vi "EEG_FFT_Analyzer.vi"() -> ()   [LabVIEW 2014]
uses:
  <vilib>/DAQmx/create/channels.llb/DAQmx Create Channel (AI-Voltage-Basic).vi
  <vilib>/DAQmx/configure/timing.llb/DAQmx Timing (Sample Clock).vi
  <vilib>/DAQmx/read.llb/DAQmx Read (Analog 1D Wfm NChan NSamp).vi
panel:
  out "Beta_Power vs. Time":dbl[](graph)
  out "Alpha_Power vs. Time":dbl[](graph)
  out "Waveform of Selected EEG":dbl[](graph)
  in  "P4":bool
  in  "P3":bool
  in  "Pz":bool
  in  "O2":bool
  in  "O1":bool
  in  "C4":bool
  in  "C3":bool
  in  "Cz":bool
  in  "F4":bool
  in  "Fz":bool
  in  "F3":bool
  in  "stop":bool
  # "NASION"
  # "INION"
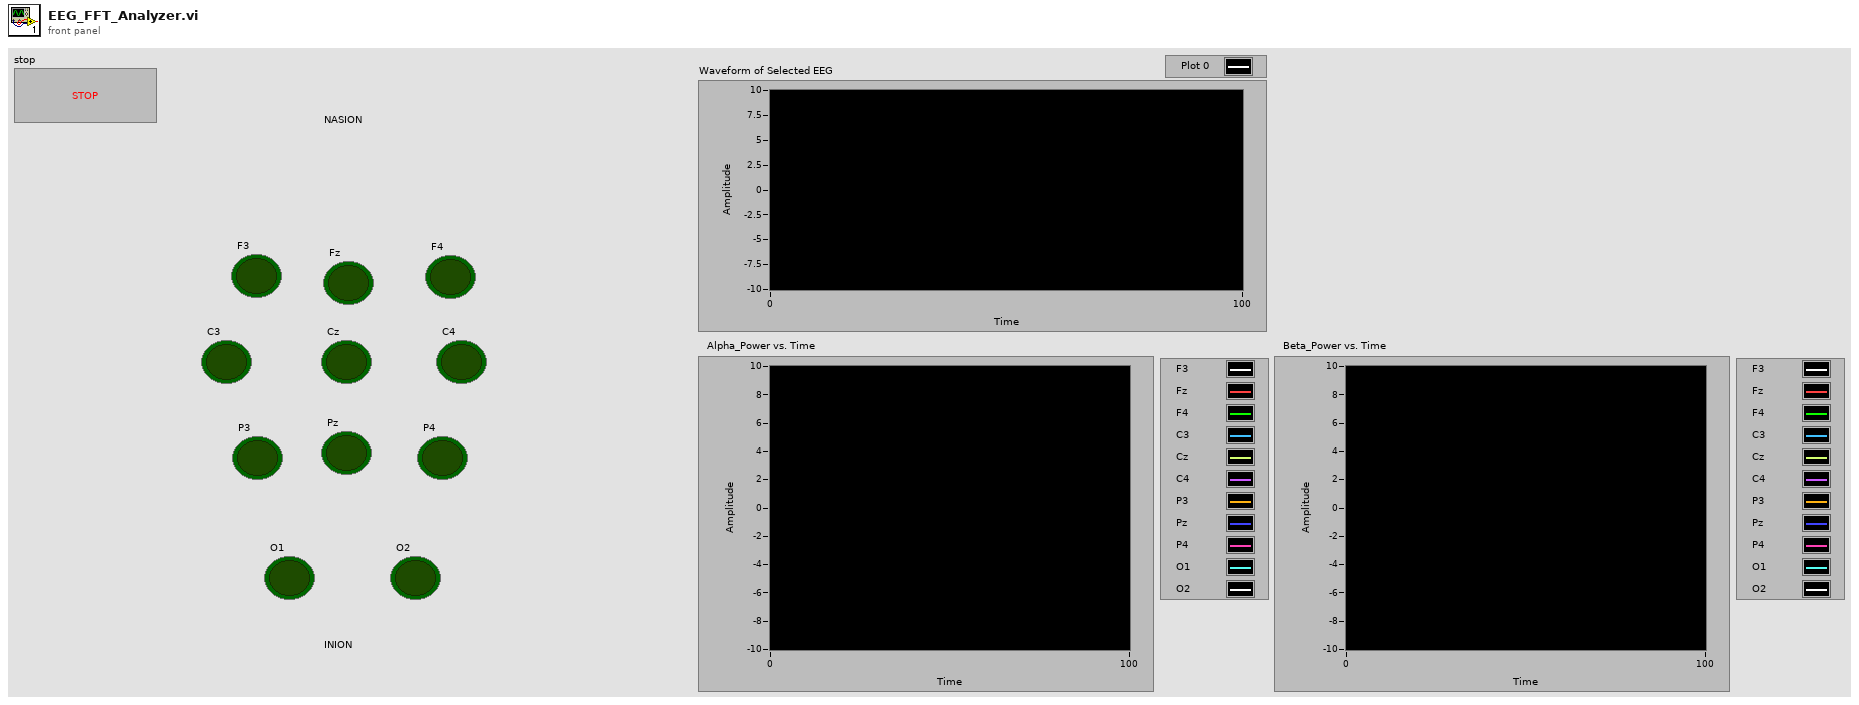
[diagram p1: front panel]
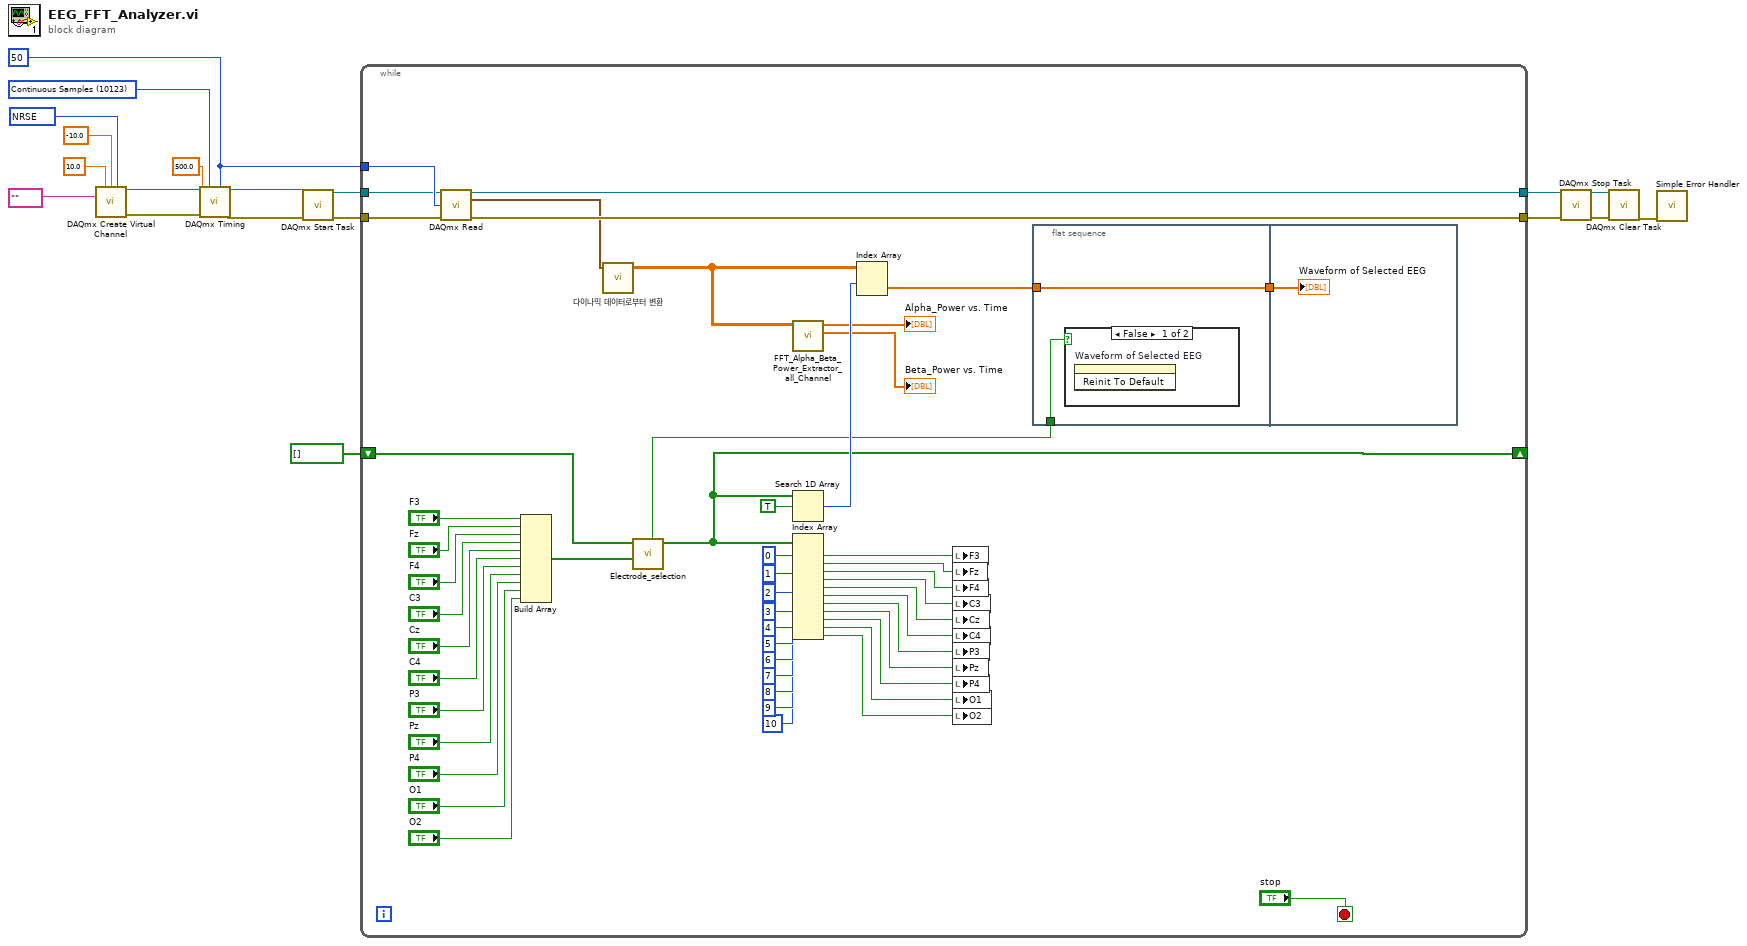
[diagram p0: block diagram]
diagram:
  w11 = 10123 items=["Finite Samples"=10178, "Continuous Samples"=10123, "Hardware Timed Single Point"=12522] ("sample mode")
  w9 = 50 ("samples per channel")
  w13 = 10078 items=["default"=-1, "RSE"=10083, "NRSE"=10078, "Differential"=10106, "Pseudodifferential"=12529] ("input terminal configuration")
  n1 = call-poly <vilib>:"DAQmx Create Virtual Channel.vi"("maximum value"=10.0, "minimum value"=-10.0, "input terminal configuration"=w13, "physical channels"=tag "") -> ("task out"=w17:refnum<k21>, "error out"=w16:errorcluster)  [unwired: 10 in]
  n2 = call-poly <vilib>:"DAQmx Timing.vi"("task/channels in"=w17, "sample mode"=w11, "samples per channel"=w9, "rate"=500.0 ("maximum value"), "error in"=w16) -> ("task out"=w15:refnum<k21>, "error out"=w14:errorcluster)  [unwired: 9 in]
  n3 = call <vilib>:"DAQmx Start Task.vi"("task/channels in"=w15, "error in"=w14) -> ("task out"=w8:refnum<k21>, "error out"=w7:errorcluster)  [unwired: 12 in]
  n4 = while {
    tunnel: w9 -> [w70]
    tunnel: w8 -> [w69]
    tunnel: w7 -> [w68]
    tunnel: [w67] -> w3
    tunnel: [w66] -> w2
    shift-right: [w26] -> _
    shift-left: bool[] [] -> [w52]
    stop <- "stop" stop-if-true
    n5 = call-poly <vilib>:"DAQmx Read.vi"("task/channels in"=w69, "number of samples per channel"=w70, "error in"=w68) -> ("task out"=w67:refnum<k21>, "data"=w65:waveform(dbl)[], "error out"=w66:errorcluster)  [unwired: 10 in]
    n6 = Build Array("F3", "Fz", "F4", "C3", "Cz", "C4", "P3", "Pz", "P4", "O1", "O2") -> (w51:bool[])
    n7 = call "다이나믹 데이터로부터 변환"("Dynamic Data Type"=w65) -> ("Array"=w25:dbl[][])  [unwired: 3 in]
    n8 = call "Electrode_selection.vi"("Array of Channel Electrodes"=w51, "Previous Channel Electrodes"=w52) -> ("Selected Electrode"=w26:bool[], "x != 0?"=w22:bool)  [unwired: 8 in]
    n9 = call "FFT_Alpha_Beta_Power_Extractor_all_Channel.vi"("NChan EEG Signal"=w25) -> ("Beta_all"=→"Beta_Power vs. Time":dbl[], "Alpha_all"=→"Alpha_Power vs. Time":dbl[])  [unwired: 9 in]
    n10 = Search 1D Array(1D array=w26, element=TRUE) -> (index of element=w27:i32)  [unwired: 1 in]
    n11 = Index Array(array=w26, index #1=0 ("index"), index #2=1 ("index"), index #3=2 ("index"), index #4=3 ("index"), index #5=4 ("index"), index #6=5 ("index"), index #7=6 ("index"), index #8=7 ("index"), index #9=8 ("index"), index #10=9 ("index"), index #11=10 ("index")) -> (element #1=w39:bool, element #2=w38:bool, element #3=w37:bool, element #4=w36:bool, element #5=w35:bool, element #6=w34:bool, element #7=w33:bool, element #8=w32:bool, element #9=w31:bool, element #10=w30:bool, element #11=w29:bool)
    n12 = Index Array(array=w25, index (row)=w27) -> (element=w21:dbl[])  [unwired: 1 in]
    n13 = local write "F3"(w39) -> ()
    n14 = local write "Fz"(w38) -> ()
    n15 = local write "F4"(w37) -> ()
    n16 = local write "C3"(w36) -> ()
    n17 = local write "Cz"(w35) -> ()
    n18 = local write "C4"(w34) -> ()
    n19 = local write "P3"(w33) -> ()
    n20 = local write "Pz"(w32) -> ()
    n21 = local write "P4"(w31) -> ()
    n22 = local write "O1"(w30) -> ()
    n23 = local write "O2"(w29) -> ()
    n24 = flat-sequence {
      tunnel: w22 -> [w72]
      tunnel: w21 -> [w71]
      tunnel: [w71] -> w20
      tunnel: w20 -> [w73]
      frame #0 {
        n25 = case shown="False" w72 {
          frame False {
            n26 = invoke on="Waveform of Selected EEG" class="WFChart (strict)" method="Reinit To Default"() -> ()  [unwired: 3 in, 3 out]
          }
          frame True {
          }
        }
      }
      frame #1 {
        "Waveform of Selected EEG" <- w73
      }
    }
  }
  n27 = call <vilib>:"DAQmx Stop Task.vi"("task/channels in"=w3, "error in"=w2) -> ("task out"=w6:refnum<k21>, "error out"=w5:errorcluster)  [unwired: 12 in]
  n28 = call <vilib>:"DAQmx Clear Task.vi"("task in"=w6, "error in"=w5) -> ("error out"=w4:errorcluster)  [unwired: 13 in]
  n29 = call <vilib>:"Simple Error Handler.vi"("error in (no error)"=w4) -> ()  [unwired: 4 in, 5 out]
